vi "Fit Zoom Picture.vi"(8 "error in (no error)":errorcluster, 10 "Images":T2[](array[typedef]), 11 "Draw Area Size":T1[](array[typedef])) -> (0 "error out":errorcluster, 2 "Images out":T2[](array[typedef]), 3 "Fit Zoom":dbl[](array[numeric]))   [LabVIEW 2014]
uses:
  <vilib>/Utility/miscctls.llb/LVBoundsTypeDef.ctl
  <vilib>/picture/picture.llb/imagedata.ctl
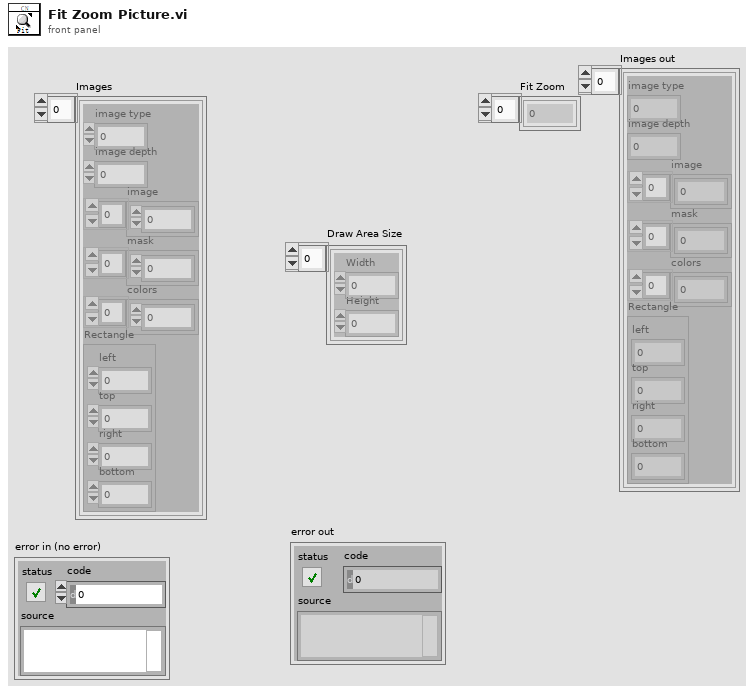
[diagram p1: front panel]
types:
  T1 = typedef "LVBoundsTypeDef.ctl" = cluster{"Width":u32, "Height":u32}
  T2 = typedef "imagedata.ctl" = cluster{"image type":i32, "image depth":i32, "image":u8[], "mask":u8[], "colors":u32[], "Rectangle":cluster{"left":i16, "top":i16, "right":i16, "bottom":i16}}
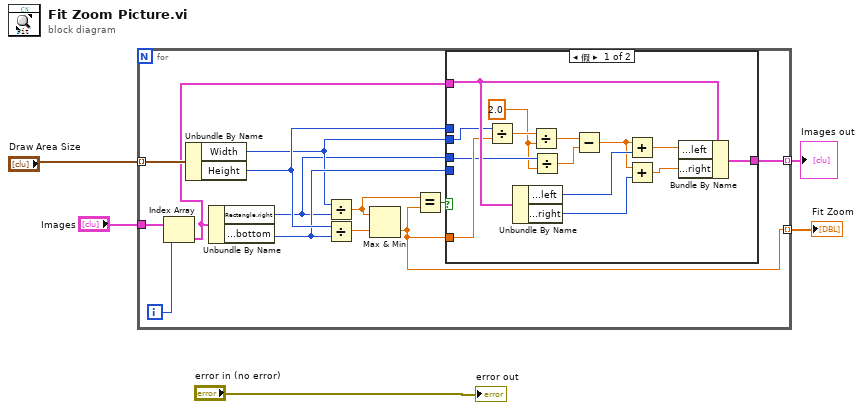
[diagram p0: block diagram]
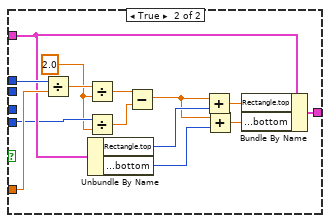
[diagram p2: hidden frame]
diagram:
  n1 = for {
    tunnel: "Images" -> [w8]
    tunnel: "Draw Area Size" -> [w18] mode=indexing
    tunnel: [w10] -> w3 mode=indexing
    tunnel: [w9] -> w2 mode=indexing
    i -> [w6]
    n2 = Index Array(array=w8, index=w6) -> (element=w7:T2)
    n3 = Unbundle By Name(w18) -> ("Width"=w12:u32, "Height"=w14:u32)
    n4 = Unbundle By Name(w7) -> ("Rectangle.right"=w11:i16, "Rectangle.bottom"=w13:i16)
    n5 = Divide(x=w12, y=w11) -> (x/y=w15:dbl)
    n6 = Divide(x=w14, y=w13) -> (x/y=w17:dbl)
    n7 = Max & Min(x=w15, y=w17) -> (min(x,y)=w10:dbl)  [unwired: 1 out]
    n8 = Equal?(x=w15, y=w10) -> (x = y?=w16:bool)
    n9 = case shown="假" w16 {
      tunnel: w14 -> [_ w46]
      tunnel: w10 -> [w29 w45]
      tunnel: w7 -> [w30 w44]
      tunnel: [w31 w43] -> w9
      tunnel: w12 -> [w28 _]
      tunnel: w11 -> [w27 _]
      tunnel: w13 -> [_ w42]
      frame False {
        w26 = 2.0 ("y")
        n10 = Divide(x=w28, y=w29) -> (x/y=w32:dbl)
        n11 = Unbundle By Name(w30) -> ("Rectangle.left"=w23:i16, "Rectangle.right"=w19:i16)
        n12 = Divide(x=w32, y=w26) -> (x/y=w25:dbl)
        n13 = Divide(x=w27, y=w26) -> (x/y=w24:dbl)
        n14 = Subtract(x=w25, y=w24) -> (x-y=w20:dbl)
        n15 = Add(x=w20, y=w23) -> (x+y=w22:dbl)
        n16 = Add(x=w20, y=w19) -> (x+y=w21:dbl)
        n17 = Bundle By Name(cluster=w30, "Rectangle.left"=w22, "Rectangle.right"=w21) -> (w31:T2)
      }
      frame True {
        w40 = 2.0 ("y")
        n18 = Divide(x=w46, y=w45) -> (x/y=w41:dbl)
        n19 = Divide(x=w41, y=w40) -> (x/y=w39:dbl)
        n20 = Divide(x=w42, y=w40) -> (x/y=w33:dbl)
        n21 = Unbundle By Name(w44) -> ("Rectangle.top"=w37:i16, "Rectangle.bottom"=w35:i16)
        n22 = Subtract(x=w39, y=w33) -> (x-y=w36:dbl)
        n23 = Add(x=w36, y=w37) -> (x+y=w38:dbl)
        n24 = Add(x=w36, y=w35) -> (x+y=w34:dbl)
        n25 = Bundle By Name(cluster=w44, "Rectangle.top"=w38, "Rectangle.bottom"=w34) -> (w43:T2)
      }
    }
  }
  "Fit Zoom" <- w3
  "Images out" <- w2
  "error out" <- "error in (no error)"
